vi "PH_Waveplate-GUI_6P.set i Attr.vi"(3 "error in (no error)":errorcluster, 5 "Instance Name":string) -> (0 "error out":errorcluster, 1 "i Attributes":T1 {"Type" items=["Degrees", "Percent"]}, 2 "Default Type":T2 items=["Degrees", "Percent"])   [LabVIEW 2014, in "PH_Waveplate-GUI_6P.lvlib"]
doc: "This VI reads the DB special 0 and 1 DB entries which are the axis names and writes them to own attributes. Depending on this, several GUI elements are set."
uses:
  PH_Waveplate-GUI_6P.lvlib
  PH_Waveplate-GUI_6P.Type.ctl
  PH_Waveplate-GUI_6P.i attribute.ctl
  PH_Basics/PH_Common/PH_Common.lvlib
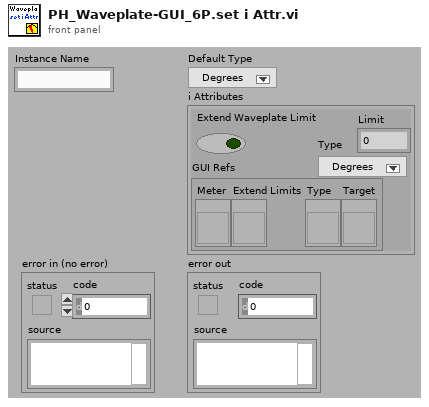
[diagram p1: front panel]
types:
  T1 = typedef "PH_Waveplate-GUI_6P.lvlib/PH_Waveplate-GUI_6P.i attribute.ctl" = cluster{"GUI Refs":cluster{"Meter":refnum<vi>, "Extend Limits":refnum<vi>, "Type":refnum<vi>, "Target":refnum<vi>}, "Extend Waveplate Limit":bool, "Type":T2, "Limit":dbl}
  T2 = typedef "PH_Waveplate-GUI_6P.lvlib/PH_Waveplate-GUI_6P.Type.ctl" = u16
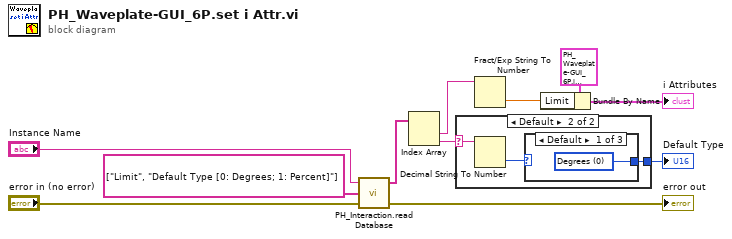
[diagram p0: block diagram]
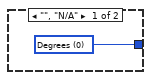
[diagram p2: hidden frame]
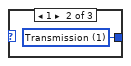
[diagram p3: hidden frame]
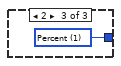
[diagram p4: hidden frame]
diagram:
  n1 = call "PH_Interaction.read Database.vi"("error in (no error)"="error in (no error)", "Strings to search for"=string[] ["Limit", "Default Type [0: Degrees; 1: Percent]"] ("Strings to search for in"), "DB Entry to read"="Instance Name") -> ("error out"=→"error out":errorcluster, "Values"=w6:string[])  [unwired: 1 in]
  n2 = Index Array(array=w6) -> (element #1=w5:string, element #2=w4:string)  [unwired: 2 in]
  n3 = case shown="Default" w4 {
    selector: w4 -> [_ w15]
    tunnel: [w12 w13] -> w10
    frame "", "N/A" {
      w12 = T2 0 items=["Degrees", "Percent"] ("Type")
    }
    frame Default {
      n4 = Decimal String To Number(string=w15) -> (number=w14:i32)  [unwired: 2 in, 1 out]
      n5 = case shown="Default" w14 {
        tunnel: [w16 w17 w18] -> w13
        frame Default {
          w16 = T2 0 items=["Degrees", "Percent"] ("Type")
        }
        frame 1 {
          w17 = T2 1 items=["Normal", "Transmission", "Reflection"] ("Type")
        }
        frame 2 {
          w18 = T2 1 items=["Degrees", "Percent"] ("Type")
        }
      }
    }
  }
  "Default Type" <- w10
  n6 = Fract/Exp String To Number(string=w5) -> (number=w2:dbl)  [unwired: 3 in, 1 out]
  n7 = Bundle By Name(cluster=T1 {"GUI Refs"={"Meter"=refnum, "Extend Limits"=refnum, "Type"=refnum, "Target"=refnum}, "Extend Waveplate Limit"=FALSE, "Type"=0, "Limit"=0.0} ("CLASS.i attribute"), "Limit"=w2) -> (→"i Attributes":T1)
